vi "Main_Fun_Controls Enable.vi"(7 "Controls Action":T1(ring), 9 "Control Name Array In":string[](array[string]), 10 "Controls In":refnum<vi>[](array[refnum]), 11 "This VI Reference":refnum<vi>) -> ()   [LabVIEW 2015]
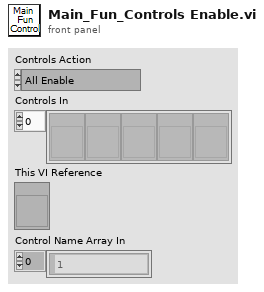
[diagram p1: front panel]
types:
  T1 = enum16{"All Enable", "All Disable", "Port Enable", "Port Disable"}
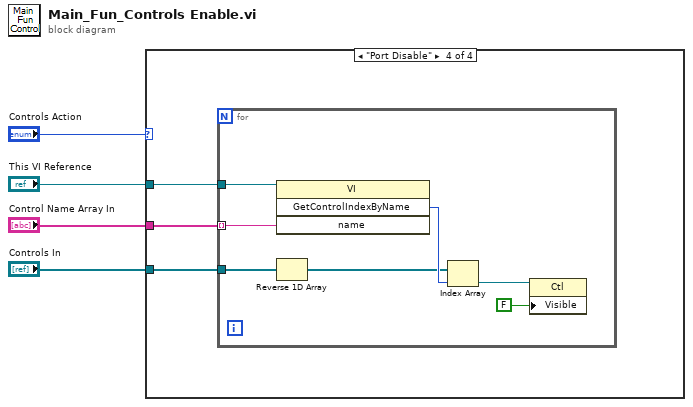
[diagram p0: block diagram]
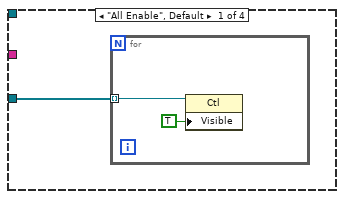
[diagram p2: hidden frame]
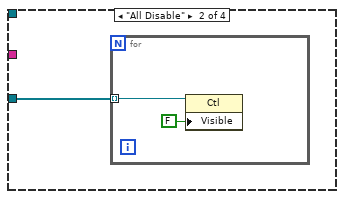
[diagram p3: hidden frame]
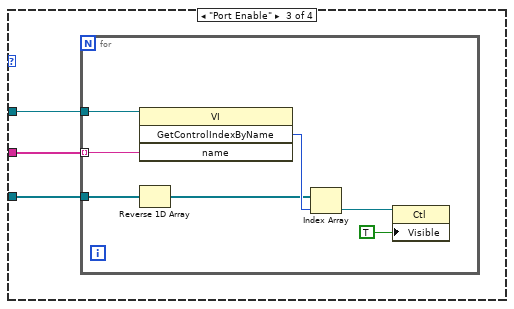
[diagram p4: hidden frame]
diagram:
  n1 = case shown="\"Port Disable\"" "Controls Action" {
    tunnel: "This VI Reference" -> [_ _ w12 w22]
    tunnel: "Control Name Array In" -> [_ _ w13 w21]
    tunnel: "Controls In" -> [w5 w8 w11 w23]
    frame "All Enable", Default {
      n2 = for {
        tunnel: w5 -> [w6] mode=indexing
        n3 = property class="Ctl"(reference=w6, "Visible"=TRUE) -> ()  [unwired: 1 in, 2 out]
      }
    }
    frame "All Disable" {
      n4 = for {
        tunnel: w8 -> [w9] mode=indexing
        n5 = property class="Ctl"(reference=w9, "Visible"=FALSE) -> ()  [unwired: 1 in, 2 out]
      }
    }
    frame "Port Enable" {
      n6 = for {
        tunnel: w13 -> [w17] mode=indexing
        tunnel: w12 -> [w16]
        tunnel: w11 -> [w15]
        n7 = invoke class="VI" method="GetControlIndexByName"(reference=w16, "name"=w17) -> ("GetControlIndexByName"=w20:i32)  [unwired: 2 in, 3 out]
        n8 = Reverse 1D Array(array=w15) -> (reversed array=w19:refnum<vi>[])
        n9 = Index Array(array=w19, index=w20) -> (element=w14:refnum<vi>)
        n10 = property class="Ctl"(reference=w14, "Visible"=TRUE) -> ()  [unwired: 1 in, 2 out]
      }
    }
    frame "Port Disable" {
      n11 = for {
        tunnel: w21 -> [w27] mode=indexing
        tunnel: w22 -> [w26]
        tunnel: w23 -> [w25]
        n12 = invoke class="VI" method="GetControlIndexByName"(reference=w26, "name"=w27) -> ("GetControlIndexByName"=w30:i32)  [unwired: 2 in, 3 out]
        n13 = Reverse 1D Array(array=w25) -> (reversed array=w29:refnum<vi>[])
        n14 = Index Array(array=w29, index=w30) -> (element=w24:refnum<vi>)
        n15 = property class="Ctl"(reference=w24, "Visible"=FALSE) -> ()  [unwired: 1 in, 2 out]
      }
    }
  }
